vi "Open Project.vi"(8 "error in (no error)":errorcluster, 11 "Editor.lvclass in":refnum<data-value>) -> (0 "error out":errorcluster, 2 "Cancelled":bool caption="cancelled", 3 "Editor.lvclass out":refnum<data-value>)   [LabVIEW 2015, in "Editor.lvclass"]
uses:
  Editor.lvclass
  Project.lvclass
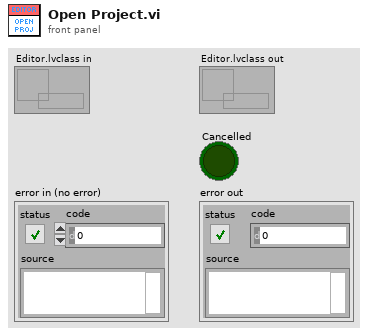
[diagram p1: front panel]
types:
  T1 = enum16{"Left Button", "Center Button", "Right Button", "Window Close"}
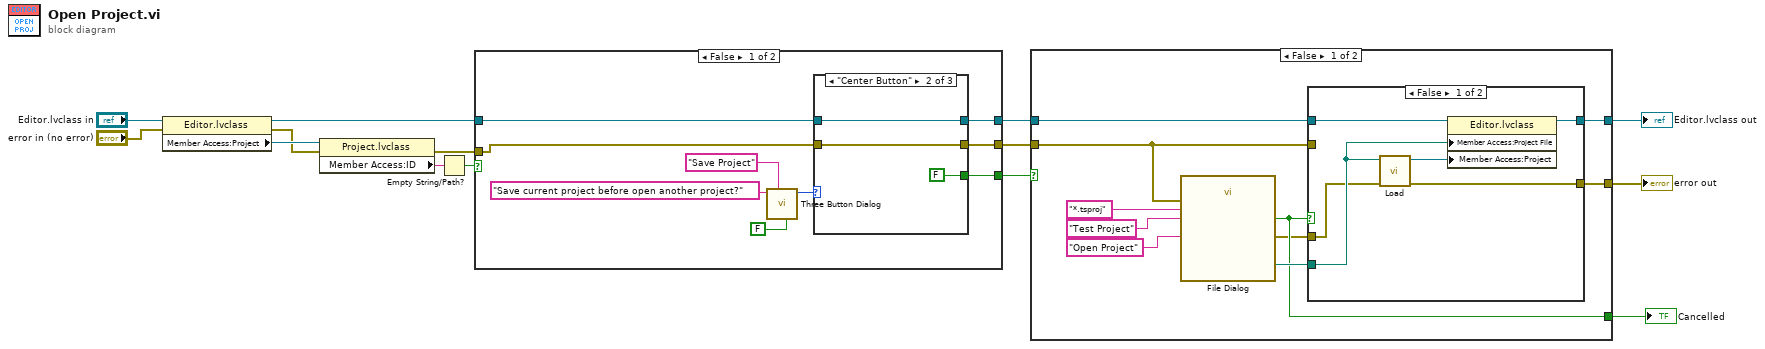
[diagram p0: block diagram]
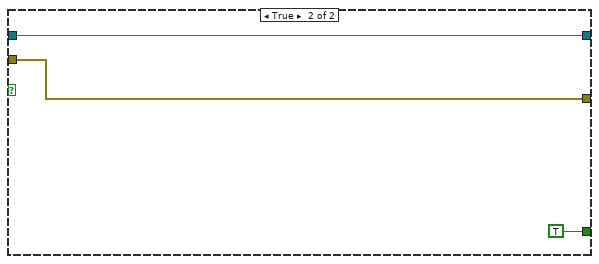
[diagram p3: hidden frame]
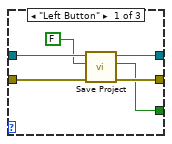
[diagram p4: hidden frame]
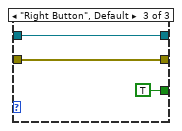
[diagram p5: hidden frame]
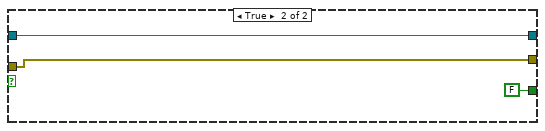
[diagram p6: hidden frame]
diagram:
  n1 = property class="Editor.lvclass"(reference="Editor.lvclass in", error in="error in (no error)") -> (reference out=w7:refnum<data-value>, error out=w9:errorcluster, "Member Access:Project"=w11:refnum<class "Project.lvclass">)
  n2 = property class="Project.lvclass"(reference=w11, error in=w9) -> (error out=w6:errorcluster, "Member Access:ID"=w10:string)  [unwired: 1 out]
  n3 = Empty String/Path?(string/path=w10) -> (empty?=w8:bool)
  n4 = case shown="False" w8 {
    tunnel: w7 -> [w19 w38]
    tunnel: w6 -> [w18 w37]
    tunnel: [w17 w38] -> w5
    tunnel: [w16 w37] -> w4
    tunnel: [w15 FALSE] -> w1
    frame False {
      n5 = call <vilib>:"Three Button Dialog.vi"("Allow user to close window? (TRUE)"=FALSE, "Window Title (\"\")"="Save Project" ("Window Title (\"\")"), "message"="Save current project before open another project?") -> ("Which Button?"=w20:T1)  [unwired: 8 in]
      n6 = case shown="\"Center Button\"" w20 {
        tunnel: w19 -> [w29 w32 w35]
        tunnel: w18 -> [w27 w31 w34]
        tunnel: [w26 w32 w35] -> w17
        tunnel: [w25 w31 w34] -> w16
        tunnel: [w24 FALSE TRUE] -> w15
        frame "Left Button" {
          n7 = call "Save Project.vi"("error in (no error)"=w27, "Save As"=FALSE, "Editor.lvclass in"=w29) -> ("error out"=w25:errorcluster, "Cancelled"=w24:bool, "Editor.lvclass out"=w26:refnum<data-value>)  [unwired: 6 in]
        }
        frame "Center Button" {
        }
        frame "Right Button", Default {
        }
      }
    }
    frame True {
    }
  }
  n8 = case shown="False" w1 {
    tunnel: [w48 w58] -> w14
    tunnel: [w47 w57] -> w13
    tunnel: [w42 TRUE ("cancelled")] -> w12
    tunnel: w5 -> [w40 w58]
    tunnel: w4 -> [w39 w57]
    frame False {
      n9 = call "File Dialog"("prompt"="Open Project", "error in"=w39, "pattern (all files)"="*.tsproj" ("pattern label"), "pattern label"="Test Project" ("button label")) -> ("selected path"=w46:path, "cancelled"=w42:bool, "error out"=w41:errorcluster)  [unwired: 8 in, 1 out]
      n10 = case shown="False" w42 {
        tunnel: [w54 w56] -> w48
        tunnel: w40 -> [w53 w56]
        tunnel: [w49 w55] -> w47
        tunnel: w46 -> [w52 _]
        tunnel: w41 -> [w51 _]
        tunnel: w39 -> [_ w55]
        frame False {
          n11 = call "Load.vi"("error in (no error)"=w51, "Project File"=w52) -> ("error out"=w49:errorcluster, "Project"=w50:refnum<class "Project.lvclass">)  [unwired: 8 in]
          n12 = property class="Editor.lvclass"(reference=w53, "Member Access:Project File"=w52, "Member Access:Project"=w50) -> (reference out=w54:refnum<data-value>)  [unwired: 1 in, 1 out]
        }
        frame True {
        }
      }
    }
    frame True {
    }
  }
  "Editor.lvclass out" <- w14
  "error out" <- w13
  "Cancelled" <- w12
